vi "NML GPIB Bus Scan-old.vi"() -> (0 "Instrument List":T1(array[cluster]) {"Status" format="%.0x"})   [LabVIEW 2019]
doc: "Scans all primary addresses on the GPIB bus and reports status of devices found there.\nScott Hannahs, F. Bitter National Magnet Lab, April 1993"
panel:
  out "error out":errorcluster
  # "VISA Address"
  # "Status"
  # "Manufacturer"
  # "Model"
  # "Serial Number"
  # "Firmware"
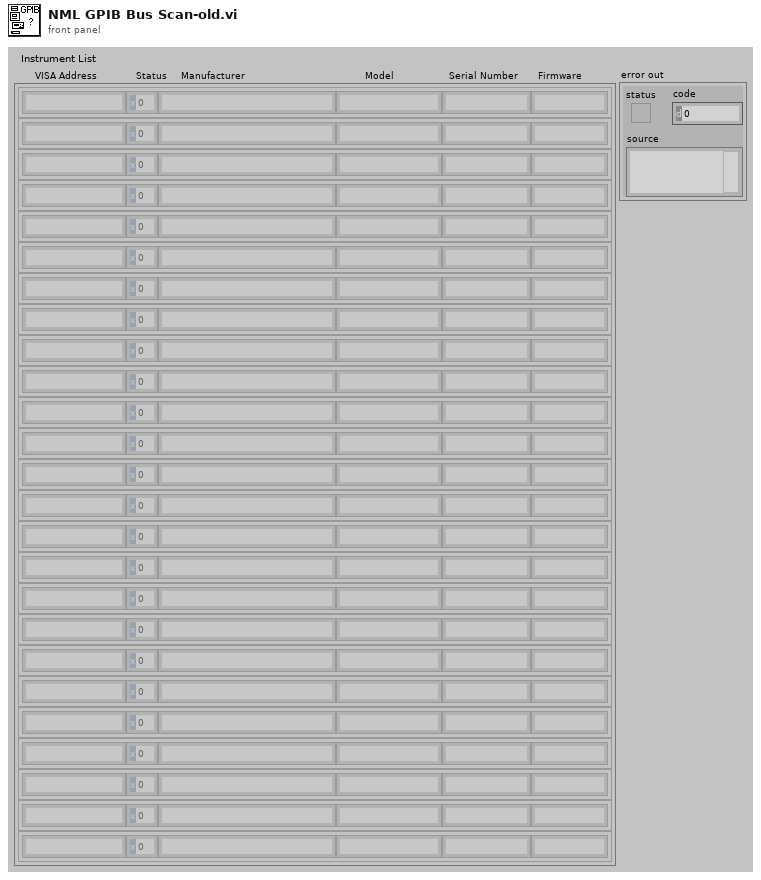
[diagram p1: front panel]
types:
  T1 = cluster{"VISA Address":string, "Status":u16, "Manufacturer":string, "Model":string, "Info":string, "Info 2":string}[]
  T2 = cluster{refnum<visa-resource-name>, "status":u16, "Manufacturer":string, "Model":string, "Info":string, "Revision":string}
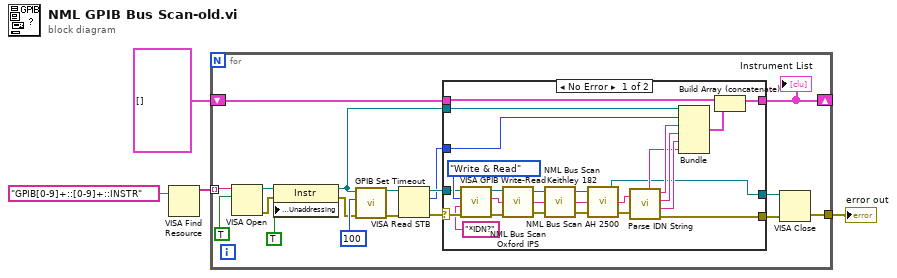
[diagram p0: block diagram]
diagram:
  n1 = VISA Find Resource(11:"GPIB[0-9]+::[0-9]+::INSTR" ("expression (\"?*\")")) -> (3:w1:string[])  [unwired: 2 in, 2 out]
  n2 = for {
    tunnel: w1 -> [w11] mode=indexing
    tunnel: [w21] -> w4
    shift-right: [w13] -> _
    shift-left: T1 [] ("Instrument List") -> [w15]
    n3 = VISA Open(duplicate session (F)=TRUE, VISA resource name=w11) -> (VISA resource name=w9:refnum<visa-resource-name>, error out=w6:errorcluster)  [unwired: 3 in]
    n4 = property class="Instr"(reference=w9, error in=w6, "GPIB Settings:Unaddressing"=TRUE ("GPIB Settings:GPIB Unaddressing")) -> (reference out=w8:refnum<visa-resource-name>, error out=w7:errorcluster)
    n5 = call "GPIB Set Timeout.vi"("Error In"=w7, "Timeout"=u32 100 ("General Settings:Timeout Value"), "VISA resource name"=w8) -> ("Error Out"=w12:errorcluster, "dup VISA resource name"=w19:refnum<visa-resource-name>)  [unwired: 2 in, 1 out]
    n6 = VISA Read STB(8:w12, 11:w19) -> (0:w16:errorcluster, 2:w14:u16, 3:w18:refnum<visa-resource-name>)
    n7 = case shown="No Error" w16 {
      selector: w16 -> [w46 w50]
      tunnel: [w34 w50] -> w22
      tunnel: w18 -> [w47 w51]
      tunnel: [w24 w51] -> w17
      tunnel: w15 -> [w41 w49]
      tunnel: [w42 w49] -> w13
      tunnel: w8 -> [w39 _]
      tunnel: w14 -> [w38 _]
      frame No Error {
        n8 = call "VISA GPIB Write-Read.vi"("error in (no error)"=w46, "Command"="*IDN?" ("write buffer (\"\")"), "Action"=enum16{"Write", "Read", "Write & Read"}."Write & Read", "VISA resource name"=w47) -> ("error out"=w44:errorcluster, "String Returned"=w43:string, "dup VISA Session"=w45:refnum<visa-resource-name>)  [unwired: 4 in, 1 out]
        n9 = call "NML Bus Scan Oxford IPS.vi"("error out"=w44, "String Read 2"=w43, "VISA session"=w45) -> ("error IO"=w33:errorcluster, "String Read"=w32:string, "VISA Resource Name"=w31:refnum<visa-resource-name>)
        n10 = call "NML Bus Scan Keithley 182.vi"("error out"=w33, "String Read In"=w32, "dup VISA session"=w31) -> ("error IO"=w27:errorcluster, "String Read Out"=w29:string, "VISA Resource Name"=w28:refnum<visa-resource-name>)
        n11 = call "NML Bus Scan AH 2500.vi"("error in (no error)"=w27, "String Read In"=w29, "VISA Session"=w28) -> ("error out"=w26:errorcluster, "String Read Out"=w25:string, "VISA Session Out"=w24:refnum<visa-resource-name>)
        n12 = call "Parse IDN String.vi"("error in (no error)"=w26, "IDN String"=w25) -> ("error out"=w34:errorcluster, "Info"=w35:string, "Model"=w36:string, "Manufacturer"=w37:string, "Revision"=w30:string)
        n13 = Bundle(w39, "status"=w38, "Manufacturer"=w37, "Model"=w36, "Info"=w35, "Revision"=w30) -> (w40:T2)  [unwired: 1 in]
        n14 = Build Array (concatenate)(w41, w40) -> (w42:T1)
      }
      frame Error {
      }
    }
    "Instrument List" <- w13
    n15 = VISA Close(VISA resource name=w17, error in (no error)=w22) -> (error out=w21:errorcluster)
  }
  "error out" <- w4
